vi "ResistanceMeasurement.vi"() -> ()   [LabVIEW 2018]
uses:
  <vilib>/MakerHub/LINX/Public/Peripherals/Digital/Digital Write N Chans.vi
  <vilib>/MakerHub/LINX/Private/Local IO/LinxDigitalWrite.vi
  <vilib>/MakerHub/LINX/Public/Utilities/Check Channel.vi
  GlobalVariables/GlobalStop.vi
  <vilib>/MakerHub/LINX/Private/Utilties/Generate Error.vi
  GlobalVariables/CurrentLevelGlobal.vi
  GlobalVariables/Voltage Level Global.vi
  <vilib>/MakerHub/LINX/LMH-LINX.lvlib
panel:
  in  "Tab Control":T1(tab)
  in  "Power Supply VISA resource name":refnum<visa-resource-name>
  in  "Serial Port for Arduino":refnum<visa-resource-name>="N/A"
  in  "SetVoltage":dbl=3.3 format="%#_13g"
  in  "Delay Time (s)":dbl=0.4
  in  "ADC Maximum Value":dbl=10.0 format="%0.2f"
  in  "ADC Minimum Value":dbl=-10.0 format="%0.2f"
  in  "ADC Sample Mode":i32(ring)=10123 items=["Finite Samples"=10178, "Continuous Samples"=10123, "Hardware Timed Single Point"=12522]
  in  "Set Max Current for FP":dbl=0.25 format="%#_13g"
  in  "ADC Sampling Rate":dbl=10000.0 format="%0.2f"
  in  "Arduino Digital Outputs":u8[](array[numeric])=[2, 3, 4, 5, 6]
  in  "Decimal Input into\nLogic Block":u8=1
  out "Beginning Time Stamp":timestamp
  out "Current output (mA)":dbl
  out "Current level\nfor output pins":dbl[](array[numeric])
  out "Ending Time Stamp 2":timestamp
  out "Binary Inputs into\nLogic Block":bool[](array[boolean])
  out "Numerical\nInput Troubleshoot":u32
  out "CurrentLevelGlobal":dbl
  out "Voltage Level Global":dbl
  out "Power Supply Error":string=" INSTRUCTIONS:\r\rNormal Use:  When using subVIs that incorporate the error in/error out (or error I/O) structure, place this handler where you want to inform the user of an error, typically at the end of the I/O data path, as the last action of the program.  If the error in error? is ERROR, the handler creates a message describing the error and its source.  If the type of dialog = 1 (default), the message is displayed to the user, who can only acknowedge it.  If the type = 2, the user can acknowledge the message or abort execution; aborting a program with active I/O is not recommended.  If the type = 0, no message is displayed; this is used to process the error programmatically, and the error out cluster elements are wired to individual terminals for that reason.  \r\rOther Use:\n\r\nlocal testing.  To test the error code of a subVI or function that does not have the error I/O structure, you can wire its error code and a source string to the local error code and error source inputs.  If error in error? indicates no error and error code is not equal to 0, the local code and source are substituted for the error in values, and error? is set TRUE (ERROR)."
  out "DAQ Error":string=" INSTRUCTIONS:\r\rNormal Use:  When using subVIs that incorporate the error in/error out (or error I/O) structure, place this handler where you want to inform the user of an error, typically at the end of the I/O data path, as the last action of the program.  If the error in error? is ERROR, the handler creates a message describing the error and its source.  If the type of dialog = 1 (default), the message is displayed to the user, who can only acknowedge it.  If the type = 2, the user can acknowledge the message or abort execution; aborting a program with active I/O is not recommended.  If the type = 0, no message is displayed; this is used to process the error programmatically, and the error out cluster elements are wired to individual terminals for that reason.  \r\rOther Use:\n\r\nlocal testing.  To test the error code of a subVI or function that does not have the error I/O structure, you can wire its error code and a source string to the local error code and error source inputs.  If error in error? indicates no error and error code is not equal to 0, the local code and source are substituted for the error in values, and error? is set TRUE (ERROR)."
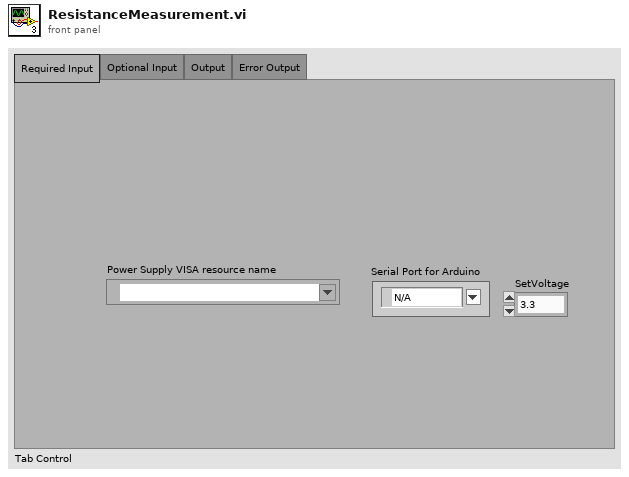
[diagram p1: front panel]
types:
  T1 = enum32{"Required Input", "Optional Input", "Output", "Error Output"}
  T2 = typedef "LMH-LINX.lvlib/LINX Ref.ctl" = cluster{"IO":T3, "Interface":T4, "LINX Device Config":T5}
  T3 = typedef "LMH-LINX.lvlib/Platform.ctl" = enum16{"Remote", "Local"}
  T4 = typedef "LMH-LINX.lvlib/Interface.ctl" = enum16{"Serial", "TCP"}
  T5 = typedef "LMH-LINX.lvlib/Device.lvlib/LINX Device Config.ctl" = cluster{"Interface":T4, "COM Port":refnum<visa-resource-name>, "TCP Configuration":T6, "Device Family":u8, "Device ID":u8, "Device Name":string, "TCP Ref":refnum<k5>, "Channels":T7}
  T6 = typedef "LMH-LINX.lvlib/Device.lvlib/TCP Config.ctl" = cluster{"IP Address":string, "Port":u16}
  T7 = typedef "LMH-LINX.lvlib/Channels.ctl" = cluster{"DI":u8[], "DO":u8[], "AI":u8[], "AO":u8[], "PWM":u8[], "QE":u8[], "UART":u8[], "I2C 2":u8[], "SPI":u8[], "CAN":u8[], "Servo":u8[], "AI Ref (V)":dbl, "AI Resolution (Bits)":u8, "AO Ref (V)":dbl, "AO Resolution (Bits)":u8}
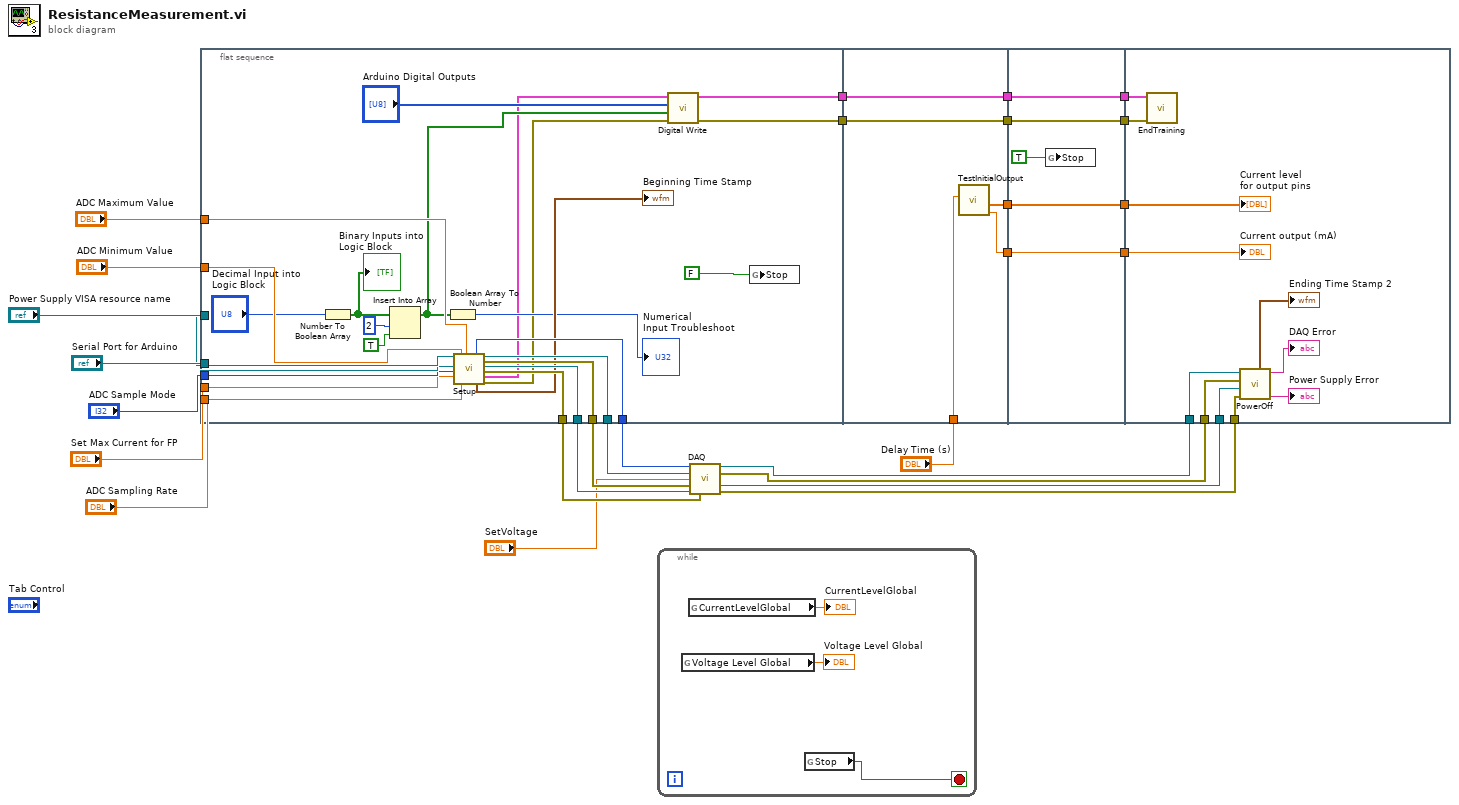
[diagram p0: block diagram]
diagram:
  n1 = flat-sequence {
    tunnel: [w53] -> w28
    tunnel: [w52] -> w27
    tunnel: [w51] -> w26
    tunnel: [w50] -> w25
    tunnel: [w49] -> w24
    tunnel: "ADC Minimum Value" -> [w47]
    tunnel: "ADC Maximum Value" -> [w46]
    tunnel: "Power Supply VISA resource name" -> [w45]
    tunnel: "Serial Port for Arduino" -> [w44]
    tunnel: "ADC Sample Mode" -> [w43]
    tunnel: "Set Max Current for FP" -> [w42]
    tunnel: "ADC Sampling Rate" -> [w41]
    tunnel: [w33] -> w11
    tunnel: [w32] -> w10
    tunnel: "Delay Time (s)" -> [w58]
    tunnel: [w57] -> w9
    tunnel: [w56] -> w7
    tunnel: [w55] -> w5
    tunnel: w11 -> [w55]
    tunnel: [w54] -> w3
    tunnel: w10 -> [w54]
    tunnel: w9 -> [w63]
    tunnel: [w63] -> w8
    tunnel: w7 -> [w62]
    tunnel: [w62] -> w6
    tunnel: w5 -> [w61]
    tunnel: [w61] -> w4
    tunnel: w3 -> [w60]
    tunnel: [w60] -> w2
    tunnel: w22 -> [w74]
    tunnel: w21 -> [w73]
    tunnel: w20 -> [w72]
    tunnel: w19 -> [w71]
    tunnel: w8 -> [w70]
    tunnel: w6 -> [w69]
    tunnel: w4 -> [w65]
    tunnel: w2 -> [w64]
    frame #0 {
      n2 = Number To Boolean Array(number="Decimal Input into\nLogic Block") -> (Boolean array=w38:bool[])
      "Binary Inputs into\nLogic Block" <- w38
      n3 = Insert Into Array(array=w38, index=2, new element=TRUE ("new element/subarray")) -> (w36:bool[])
      n4 = Boolean Array To Number(Boolean array=w36) -> (number=→"Numerical\nInput Troubleshoot":u32)
      n5 = call "Setup.vi"("Power Supply VISA resource name"=w45, "Serial Port for Arduino"=w44, "ADC Sample Mode"=w43, "Set Max Current for FP"=w42, "ADC Minimum Value"=w47, "ADC Sampling Rate"=w41, "ADC Maximum Value"=w46) -> ("Sample Length for ADC mean 2"=w49:i32, "Beginning Time Stamp"=→"Beginning Time Stamp":timestamp, "DAQ Task Out"=w53:refnum<k21>, "DAQ Error Out"=w51:errorcluster, "VISA resource name out"=w52:refnum<visa-resource-name>, "Power Supply Error Out"=w50:errorcluster, "LINX Resource"=w30:T2, "Arduino Error Out"=w31:errorcluster)  [unwired: 5 in]
      n6 = call-poly <vilib>:"Digital Write.vi"("Error In"=w31, "Values"=w36, "DO Channels"="Arduino Digital Outputs", "LINX Resource"=w30) -> ("Error Out"=w32:errorcluster, "LINX Resource"=w33:T2)  [unwired: 6 in]
      n7 = global write "GlobalStop.vi" "Stop"(FALSE ("Stop")) -> ()
    }
    frame #1 {
      n8 = call "TestInitialOutput.vi"("Delay Time (s)"=w58) -> ("Current output (mA)"=w57:dbl, "Current (mA) level\nfor output pins"=w56:dbl[])  [unwired: 8 in, 1 out]
    }
    frame #2 {
      n9 = global write "GlobalStop.vi" "Stop"(TRUE ("Stop")) -> ()
    }
    frame #3 {
      n10 = call "EndTraining.vi"("Error In"=w64, "LINX Resource"=w65) -> ()  [unwired: 10 in]
      n11 = call "PowerOff.vi"("Power Supply Error IN"=w74, "VISA resource name"=w73, "DAQ Error In"=w72, "DAQ Channels"=w71) -> ("Power Supply Error"=→"Power Supply Error":string, "DAQ Error"=→"DAQ Error":string, "Ending Time Stamp 2"=→"Ending Time Stamp 2":timestamp)  [unwired: 5 in]
      "Current output (mA)" <- w70
      "Current level\nfor output pins" <- w69
    }
  }
  n12 = while {
    stop <- w77 stop-if-true
    n13 = global read "Voltage Level Global.vi" "Voltage Level Global"() -> (→"Voltage Level Global":dbl)
    n14 = global read "CurrentLevelGlobal.vi" "CurrentLevelGlobal"() -> (→"CurrentLevelGlobal":dbl)
    n15 = global read "GlobalStop.vi" "Stop"() -> (w77:bool)
  }
  n16 = call "DAQ.vi"("sample length"=w24, "task/channels in"=w28, "SetVoltage"="SetVoltage", "error in"=w26, "VISA resource name out"=w27, "error out"=w25) -> ("task out"=w19:refnum<k21>, "error out 2"=w20:errorcluster, "VISA resource name out 2"=w21:refnum<visa-resource-name>, "error out 3"=w22:errorcluster)  [unwired: 6 in]
